vi "get array data.vi"(8 "error in (no error)":errorcluster, 11 "JSON Helper in":refnum<class "JSON Value.lvclass">) -> (0 "error out":errorcluster, 3 "JSON Array out":refnum<class "JSON Value.lvclass">[](array[class]))   [LabVIEW 2016, in "JSON Value.lvclass"]
uses:
  JSON Value.lvclass
  JSON Value.lvclass/JSON Value.ctl
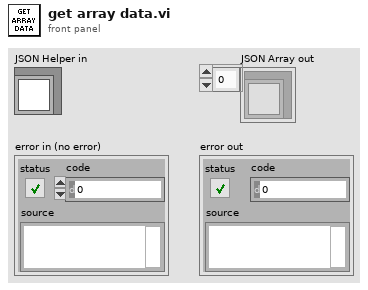
[diagram p1: front panel]
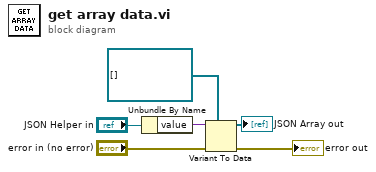
[diagram p0: block diagram]
diagram:
  n1 = Unbundle By Name("JSON Helper in") -> ("value"=w2:variant)
  n2 = Variant To Data(error in="error in (no error)", type=refnum<class "JSON Value.lvclass">[] [] ("JSON Array in"), Variant=w2) -> (data=→"JSON Array out":refnum<class "JSON Value.lvclass">[], error out=→"error out":errorcluster)
